vi "DSF.Engine.Plugin.Runtime.Set Interface.vi"(10 "Interface":refnum<class "DSF.Engine.Interface.Plugin.lvclass">, 11 "Plugin in":refnum<class "DSF.Engine.Plugin.Runtime.lvclass">) -> (3 "Plugin out":refnum<class "DSF.Engine.Plugin.Runtime.lvclass">)   [LabVIEW 2016, in "DSF.Engine.lvlib" / "DSF.Engine.Plugin.Runtime.lvclass"]
uses:
  DSF.Engine.Plugin.Runtime.lvclass
  Interface/DSF.Engine.Interface.Plugin.lvclass
  DSF.Engine.Plugin.Runtime.lvclass/DSF.Engine.Plugin.Runtime.ctl
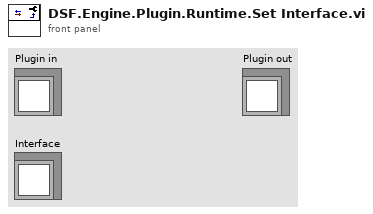
[diagram p1: front panel]
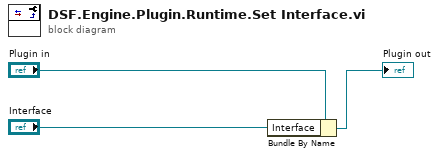
[diagram p0: block diagram]
diagram:
  n1 = Bundle By Name(cluster="Plugin in", "Interface"="Interface") -> (→"Plugin out":refnum<class "DSF.Engine.Plugin.Runtime.lvclass">)
